vi "move.vi"() -> ()   [LabVIEW 2018]
panel:
  out "appended path":path
  out "path":path
  out "filenames":string[](array[string])
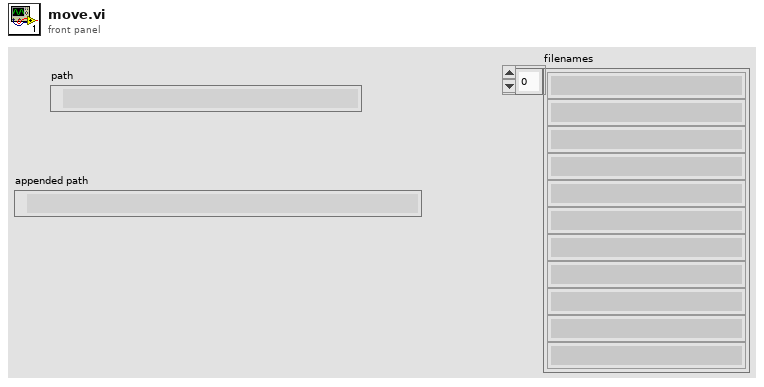
[diagram p1: front panel]
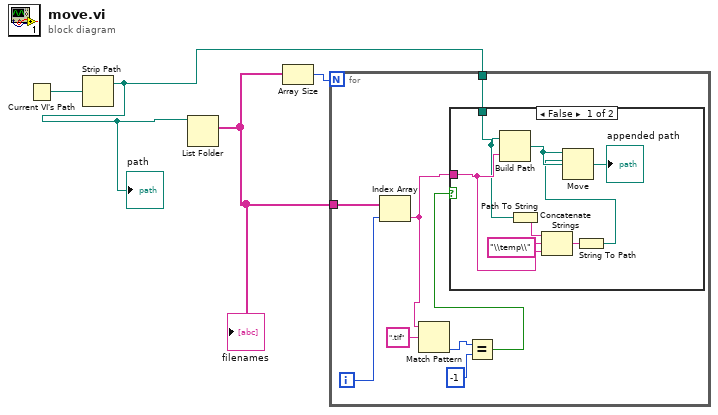
[diagram p0: block diagram]
diagram:
  n1 = Current VI's Path() -> (path=w1:path)
  n2 = Strip Path(path=w1) -> (stripped path=w2:path)  [unwired: 1 out]
  "path" <- w2
  n3 = List Folder(path=w2) -> (filenames=w3:string[])  [unwired: 3 in, 3 out]
  "filenames" <- w3
  n4 = Array Size(array=w3) -> (size(s)=w4:i32)
  n5 = for {
    N: w4 -> [_]
    tunnel: w3 -> [w12]
    tunnel: w2 -> [w5]
    i -> [w11]
    n6 = Index Array(array=w12, index=w11) -> (element=w7:string)
    n7 = Match Pattern(string=w7, regular expression=".tif") -> (offset past match=w8:i32)  [unwired: 1 in, 3 out]
    n8 = Equal?(x=w8, y=-1) -> (x = y?=w6:bool)
    n9 = case shown="False" w6 {
      tunnel: w7 -> [w14 _]
      tunnel: w5 -> [w13 _]
      frame False {
        n10 = Build Path(base path=w13, name or relative path=w14) -> (appended path=w19:path)
        "appended path" <- w19
        n11 = Path To String(path=w13) -> (string=w18:string)
        n12 = Concatenate Strings(w18, "\\temp\\", w14) -> (w16:string)
        n13 = String To Path(string=w16) -> (path=w15:path)
        n14 = Move(source path=w19, 10:w15) -> ()  [unwired: 3 in, 3 out]
      }
      frame True {
      }
    }
  }
